vi "AES DataReplay Calculate Address Multiplier.vi"(7 "CycleAngle?":bool caption="use cycle? (F)", 11 "memory size (divisible by 32)":i32) -> (2 "angle to address multiplier":fxp<+,18,7>)   [LabVIEW 2010, in "AES.lvlib" / "AES RT.lvlib"]
doc: "This VI takes the memory size for data replay and calculates the multiplier used on the FPGA to transform from angle to memory address, as well as calculates the number of memory load iterations required to load an FPGA memory of this size from the host.\n\nNote: Set the \"Use Cycle? (F)\" input to true if your Data Replay loop is referencing the Cycle Angle (0-720) not the Crank Angle (0-360)"
uses:
  AES RT.lvlib
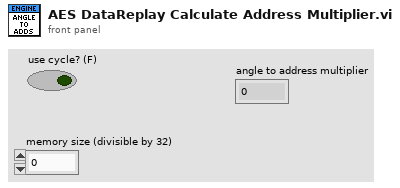
[diagram p1: front panel]
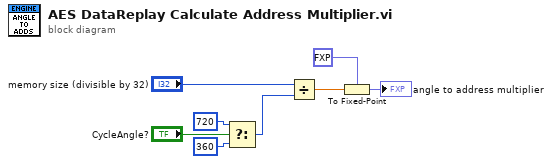
[diagram p0: block diagram]
diagram:
  n1 = Select(t=720, s="CycleAngle?", f=360) -> (s? t:f=w5:i32)
  n2 = Divide(x="memory size (divisible by 32)", y=w5) -> (x/y=w4:dbl)
  n3 = To Fixed-Point(fixed-point type=fxp<+,18,7> 0.0, number=w4) -> (fixed-point=→"angle to address multiplier":fxp<+,18,7>)
